vi "test_on_compactRIO2.vi"   [LabVIEW 2016]
uses:
  <vilib>/addons/WatchdogProcess/WatchdogProcess.lvlib
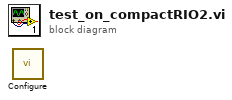
[diagram p0: block diagram]
diagram:
  n1 = call <vilib>:"Configure.vi"() -> ()  [unwired: 9 in, 3 out]
